vi "Generate Channels.vi"(8 "error in (no error)":errorcluster, 11 "references in":T1) -> (0 "error out":errorcluster)   [LabVIEW 2014, in "Scan Engine editor node.lvclass"]
uses:
  Scan Engine editor node.lvclass
  <vilib>/NI/DCAF/Tag Editor Core/Table API/Table Manager/object ref.ctl
  <vilib>/NI/DCAF/Tag Editor Core/Configuration Editor/Classes/Engine Parent/Engine Parent Editor Node.lvclass
  <vilib>/NI/DCAF/Tag Editor Core/Configuration Editor/Classes/Module editor node/module editor node.lvclass
  <vilib>/NI/Configuration Framework/serializable configuration/NISE_CEF_serializable configuration.lvclass/NISE_CEF_serializable configuration.ctl
  <vilib>/Utility/LVClass/Get LV Class Name.vi
  <vilib>/NI/Configuration Framework/error generator/NISE_error generator.vi
  configuration/Scan Engine configuration.lvclass
  <vilib>/NI/Module Execution Interface/Engine Configuration/engine configuration.lvclass
  <vilib>/NI/Configuration Framework/serializable configuration/NISE_CEF_serializable configuration.lvclass
  <vilib>/NI/Tag Bus Module Framework/channel/TBM channel.lvclass
  <vilib>/NI/DCAF/Tag Editor Core/Table API/Table Manager/Table Manager.lvclass
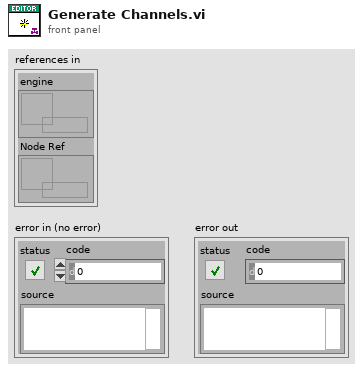
[diagram p1: front panel]
types:
  T1 = typedef "Table Manager.lvlib/Table Manager.lvclass/object ref.ctl" = cluster{"engine":refnum<data-value>, "Node Ref":refnum<data-value>}
  T2 = typedef "TBM channel.lvclass/channel classification.ctl" = enum16{"input data", "output data", "processing parameter", "processing result"}
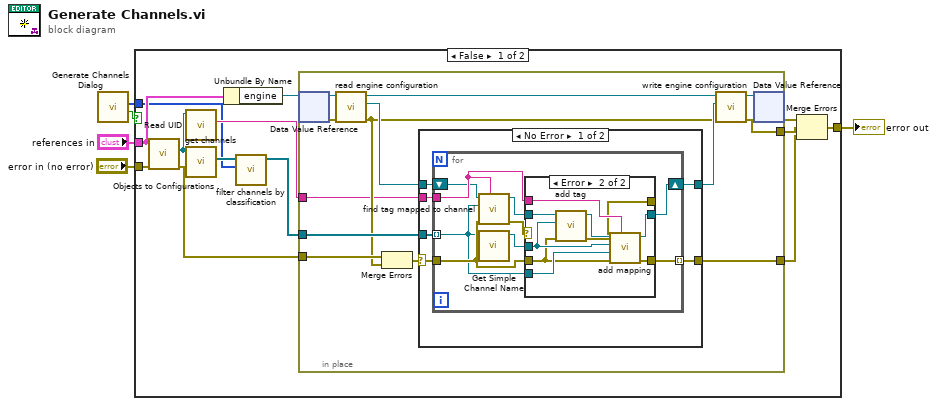
[diagram p0: block diagram]
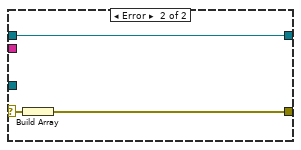
[diagram p3: hidden frame]
diagram:
  n1 = call "Generate Channels Dialog.vi"() -> ("Cancel Out"=w2:bool, "allowed classifications"=w1:T2[])  [unwired: 10 in]
  n2 = case shown="False" w2 {
    tunnel: [w15 w61] -> w5
    tunnel: "references in" -> [w12 _]
    tunnel: "error in (no error)" -> [w10 w61]
    tunnel: w1 -> [w6 _]
    frame False {
      n3 = call "Objects to Configurations.vi"("error in (no error)"=w10, "Objects in"=w12) -> ("error out"=w9:errorcluster, "tag bus configurable plugin module configuration"=w11:refnum<class "Scan Engine configuration.lvclass">)  [unwired: 7 in, 1 out]
      n4 = call <vilib>:"Read UID.vi"("configuration in"=w11) -> ("instance id"=w18:string)  [unwired: 8 in, 2 out]
      n5 = call-dynamic "get channels.vi"("Scan Engine configuration in"=w11) -> ("channels"=w8:refnum<class "TBM channel.lvclass">[])  [unwired: 9 in, 1 out]
      n6 = Unbundle By Name(w12) -> ("engine"=w13:refnum<data-value>)
      n7 = call <vilib>:"filter channels by classification.vi"("allowed classifications"=w6, "channels in"=w8) -> ("channels out"=w7:refnum<class "TBM channel.lvclass">[])  [unwired: 9 in]
      n8 = in-place {
        in-place-border: [w31] -> w14
        in-place-border: w9 -> [w30]
        in-place-border: w7 -> [w29]
        in-place-border: [w20] -> w16
        in-place-border: w18 -> [w19]
        n9 = in-place-dvr #1(w13) -> (w28:refnum<class "Engine Parent Editor Node.lvclass">, w27:errorcluster)
        n10 = call <vilib>:"read engine configuration.vi"("error in"=w27, "Engine Parent Editor Node in"=w28) -> ("error out"=w22:errorcluster, "engine configuration"=w23:refnum<class "engine configuration.lvclass">, "Engine Parent Editor Node out"=w26:refnum<class "Engine Parent Editor Node.lvclass">)  [unwired: 7 in]
        n11 = Merge Errors(w30, w22) -> (w21:errorcluster)
        n12 = case shown="No Error" w21 {
          selector: w21 -> [w33 w59]
          tunnel: [w37 w58] -> w31
          tunnel: w29 -> [w36 _]
          tunnel: [w35 w60] -> w24
          tunnel: w23 -> [w34 w60]
          tunnel: w19 -> [w32 _]
          frame No Error {
            n13 = for {
              tunnel: w36 -> [w38] mode=indexing
              shift-right: [w46] -> w35
              shift-left: w34 -> [w42]
              tunnel: w33 -> [w44]
              tunnel: [w45] -> w37 mode=indexing
              tunnel: w32 -> [w43]
              n14 = call <vilib>:"find tag mapped to channel.vi"("owner"=w43, "error in"=w44, "channel"=w38, "engine configuration in"=w42) -> ("error out"=w40:errorcluster, "engine configuration out"=w41:refnum<class "engine configuration.lvclass">)  [unwired: 5 in, 1 out]
              n15 = call "Get Simple Channel Name.vi"("channel"=w38) -> ("channel 2"=w39:refnum<class "TBM channel.lvclass">)  [unwired: 10 in]
              n16 = case shown="Error" w40 {
                selector: w40 -> [w47 _]
                tunnel: [w48 w56] -> w46
                tunnel: [w47 w55] -> w45
                tunnel: w43 -> [_ w54]
                tunnel: w39 -> [_ w53]
                tunnel: w41 -> [w48 w52]
                tunnel: w44 -> [_ w49]
                tunnel: w38 -> [_ w51]
                tunnel: [_ w50] -> _
                frame No Error {
                }
                frame Error {
                  n17 = call-dynamic "add tag.vi"("error in"=w49, "tag descriptor"=w53, "engine configuration in"=w52) -> ("error out"=w50:errorcluster, "engine configuration out"=w57:refnum<class "engine configuration.lvclass">)  [unwired: 7 in]
                  n18 = call-dynamic "add mapping.vi"("owner ID"=w54, "error in"=w49, "channel"=w51, "tag descriptor"=w53, "engine configuration"=w57) -> ("error out"=w55:errorcluster, "engine configuration out"=w56:refnum<class "engine configuration.lvclass">)  [unwired: 5 in]
                }
              }
            }
          }
          frame Error {
            n19 = Build Array(w59) -> (w58:errorcluster[])
          }
        }
        n20 = call <vilib>:"write engine configuration.vi"("error in"=w22, "engine configuration"=w24, "Engine Parent Editor Node in"=w26) -> ("error out"=w20:errorcluster, "Engine Parent Editor Node out"=w25:refnum<class "Engine Parent Editor Node.lvclass">)  [unwired: 7 in]
        n21 = in-place-dvr #1(w25) -> (w17:errorcluster)  [unwired: 1 out]
      }
      n22 = Merge Errors(w17, w16, w14) -> (w15:errorcluster)
    }
    frame True {
    }
  }
  "error out" <- w5
